vi "MeasureAndStep.vi"(4 "CC (1)/VC (0)":bool, 6 "Last Current/Voltage Value (0 A/V)":dbl, 8 "error in (no error)":errorcluster, 9 "Current/Voltage Step (0 A/V)":dbl, 10 "End Current/Voltage [A/V]":dbl, 11 "VISA resource name":refnum<visa-resource-name>) -> (0 "error out":errorcluster, 1 "CURR":dbl, 2 "VOLT":dbl, 3 "VISA resource name out":refnum<visa-resource-name>)   [LabVIEW 2017]
panel:
  out "read buffer":string
  out "resulting string":string
  out "x+y":dbl
  # "Output probes, use for debugging."
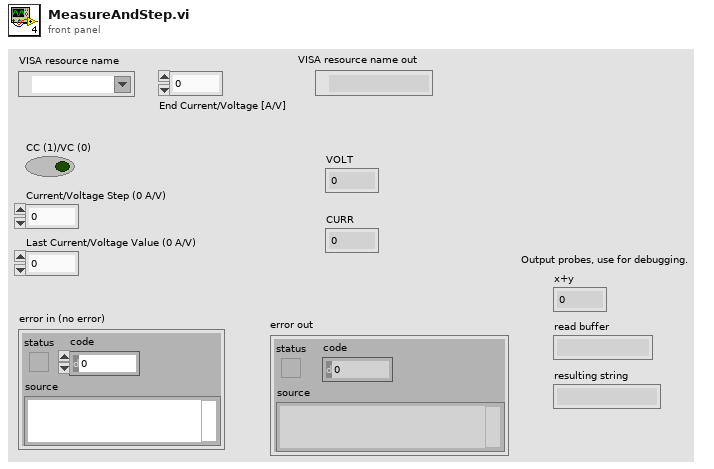
[diagram p1: front panel]
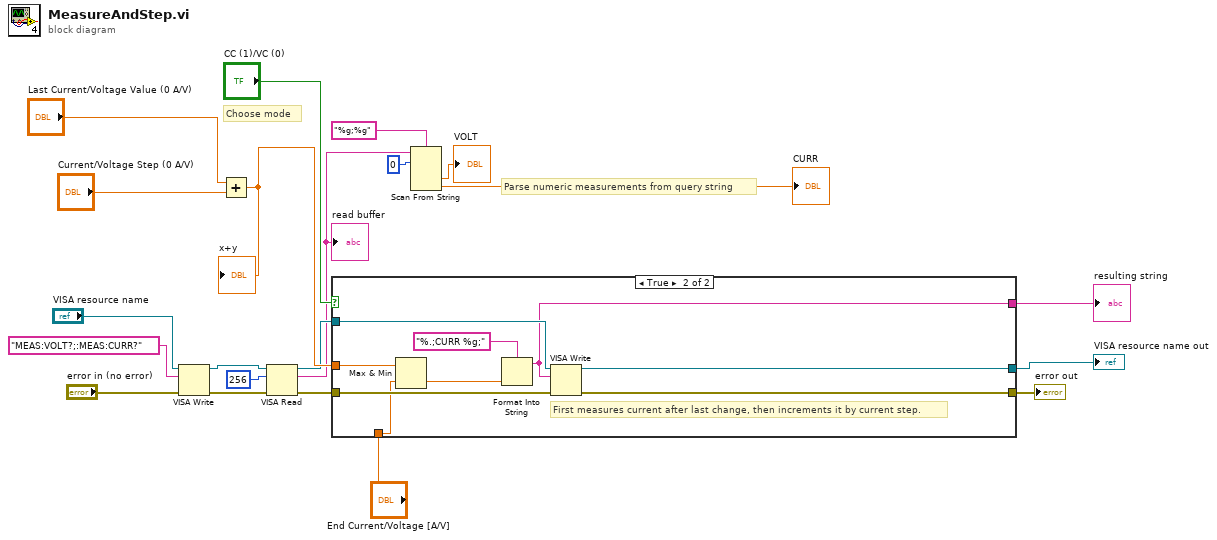
[diagram p0: block diagram]
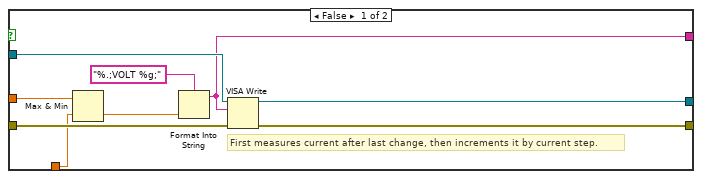
[diagram p2: hidden frame]
diagram:
  # "Choose mode"
  # "Parse numeric measurements from query string"
  n1 = VISA Write(VISA resource name="VISA resource name", write buffer="MEAS:VOLT?;:MEAS:CURR?", error in (no error)="error in (no error)") -> (VISA resource name out=w10:refnum<visa-resource-name>, error out=w9:errorcluster)  [unwired: 1 out]
  n2 = Add(x="Last Current/Voltage Value (0 A/V)", y="Current/Voltage Step (0 A/V)") -> (x+y=w14:dbl)
  "x+y" <- w14
  n3 = VISA Read(VISA resource name=w10, byte count=u32 256, error in (no error)=w9) -> (VISA resource name out=w13:refnum<visa-resource-name>, read buffer=w4:string, error out=w12:errorcluster)  [unwired: 1 out]
  "read buffer" <- w4
  n4 = case shown="True" "CC (1)/VC (0)" {
    tunnel: w14 -> [w25 w35]
    tunnel: [w23 w32] -> w18
    tunnel: [w22 w31] -> w17
    tunnel: w13 -> [w29 w38]
    tunnel: w12 -> [w28 w37]
    tunnel: [w27 w36] -> w2
    tunnel: "End Current/Voltage [A/V]" -> [w26 w34]
    frame False {
      # "First measures current after last change, then increments it by current step."
      n5 = Max & Min(x=w25, y=w26) -> (min(x,y)=w24:dbl)  [unwired: 1 out]
      n6 = Format Into String(format string="%.;VOLT %g;", w24) -> (resulting string=w27:string)  [unwired: 2 in, 1 out]
      n7 = VISA Write(VISA resource name=w29, write buffer=w27, error in (no error)=w28) -> (VISA resource name out=w23:refnum<visa-resource-name>, error out=w22:errorcluster)  [unwired: 1 out]
    }
    frame True {
      # "First measures current after last change, then increments it by current step."
      n8 = Max & Min(x=w35, y=w34) -> (min(x,y)=w33:dbl)  [unwired: 1 out]
      n9 = Format Into String(format string="%.;CURR %g;", w33) -> (resulting string=w36:string)  [unwired: 2 in, 1 out]
      n10 = VISA Write(VISA resource name=w38, write buffer=w36, error in (no error)=w37) -> (VISA resource name out=w32:refnum<visa-resource-name>, error out=w31:errorcluster)  [unwired: 1 out]
    }
  }
  "VISA resource name out" <- w18
  "error out" <- w17
  "resulting string" <- w2
  n11 = Scan From String(format string="%g;%g", input string=w4, initial scan location=u32 0) -> (output 1=→"VOLT":dbl, output 2=→"CURR":dbl)  [unwired: 3 in, 3 out]
